vi "GetInputPads.vi"(8 "Error In":errorcluster, 11 "Pattern Node In":refnum<k20>) -> (0 "Error Out":errorcluster, 2 "Inputs":T1[](array[typedef]), 3 "Pattern Node Out":refnum<k20>)   [LabVIEW 2012, in "Virtual-PGA.lvlib"]
uses:
  Virtual-PGA.lvlib
  Public/Controls/Input.ctl
  <vilib>/xml/NI_XML.lvlib
  <resource>/objmgr/DOMUserDefRef.rc
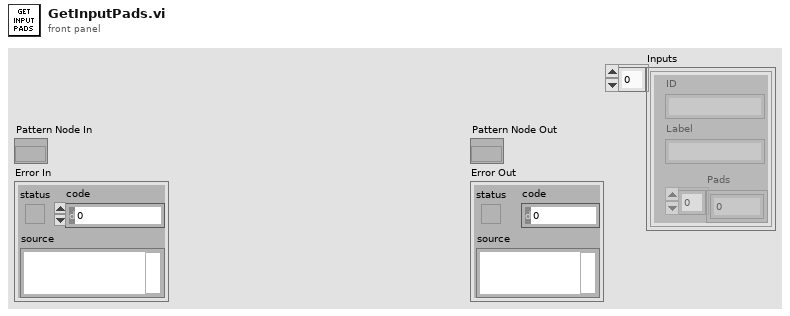
[diagram p1: front panel]
types:
  T1 = typedef "Virtual-PGA.lvlib/Input.ctl" = cluster{"ID":string, "Label":string, "Pads":u32[]}
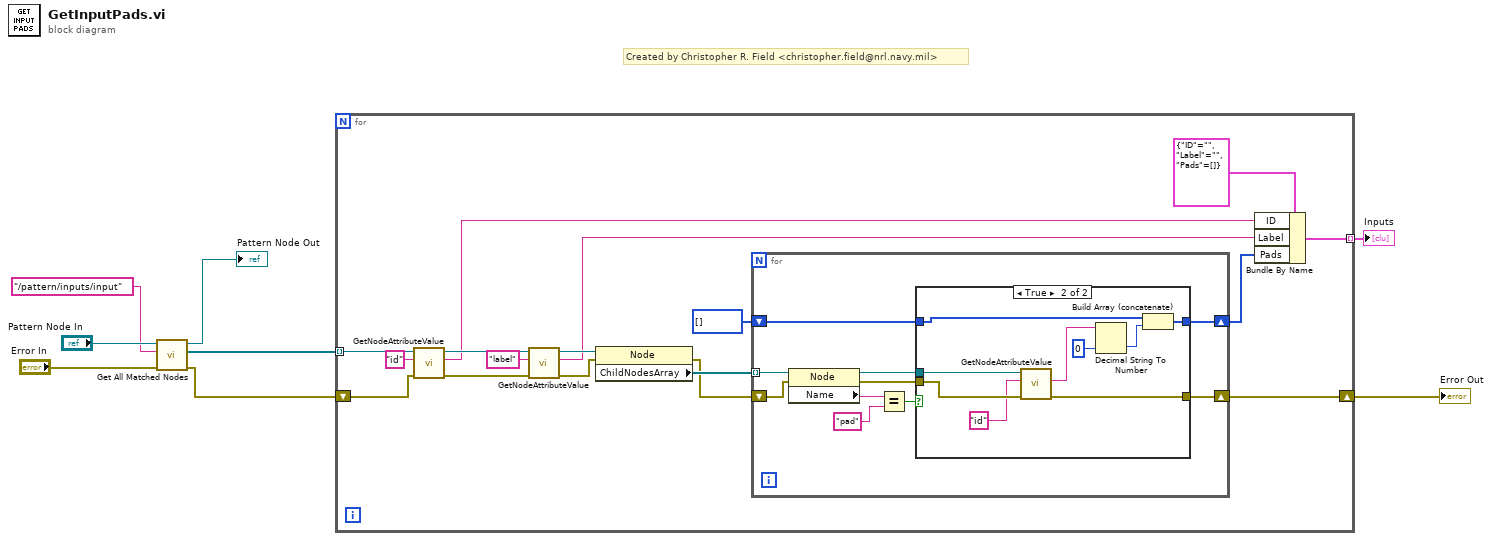
[diagram p0: block diagram]
diagram:
  # "Created by Christopher R. Field <christopher.field@nrl.navy.mil>"
  n1 = call <vilib>:"Get All Matched Nodes.vi"("error in (no error)"="Error In", "XPath expression"="/pattern/inputs/input", "node in"="Pattern Node In") -> ("error out"=w4:errorcluster, "node result array"=w3:refnum<k20>[], "node out"=→"Pattern Node Out":refnum<k20>)  [unwired: 6 in]
  n2 = for {
    tunnel: w3 -> [w23] mode=indexing
    tunnel: [w11] -> w2 mode=indexing
    shift-right: [w9] -> w1
    shift-left: w4 -> [w22]
    n3 = call "GetNodeAttributeValue.vi"("Error In"=w22, "Attribute Name"="id", "Node In"=w23) -> ("Error Out"=w18:errorcluster, "Value"=w15:string, "Node Out"=w20:refnum<k20>)  [unwired: 6 in]
    n4 = call "GetNodeAttributeValue.vi"("Error In"=w18, "Attribute Name"="label", "Node In"=w20) -> ("Error Out"=w10:errorcluster, "Value"=w14:string, "Node Out"=w19:refnum<k20>)  [unwired: 6 in]
    n5 = property class="Node"(reference=w19, error in=w10) -> (error out=w24:errorcluster, "ChildNodesArray"=w25:refnum<k20>[])  [unwired: 1 out]
    n6 = for {
      tunnel: w25 -> [w35] mode=indexing
      shift-right: [w28] -> w12
      shift-left: u32[] [] -> [w27]
      shift-right: [w26] -> w9
      shift-left: w24 -> [w34]
      n7 = property class="Node"(reference=w35, error in=w34) -> (reference out=w30:refnum<k20>, error out=w29:errorcluster, "Name"=w33:string)
      n8 = Equal?(x=w33, y="pad") -> (x = y?=w31:bool)
      n9 = case shown="True" w31 {
        tunnel: w30 -> [_ w46]
        tunnel: w29 -> [w36 w45]
        tunnel: [w37 w41] -> w28
        tunnel: w27 -> [w37 w40]
        tunnel: [w36 w38] -> w26
        frame False {
        }
        frame True {
          n10 = call "GetNodeAttributeValue.vi"("Error In"=w45, "Attribute Name"="id", "Node In"=w46) -> ("Error Out"=w38:errorcluster, "Value"=w43:string)  [unwired: 6 in, 1 out]
          n11 = Decimal String To Number(string=w43, default (0L)=u32 0) -> (number=w42:u32)  [unwired: 1 in, 1 out]
          n12 = Build Array (concatenate)(w40, w42) -> (w41:u32[])
        }
      }
    }
    n13 = Bundle By Name(cluster=T1 {"ID"="", "Label"="", "Pads"=[]} ("Input"), "ID"=w15, "Label"=w14, "Pads"=w12) -> (w11:T1)
  }
  "Error Out" <- w1
  "Inputs" <- w2
